vi "Connect.vi"(8 "error in (no error)":errorcluster, 9 "SQLITE3 open flags":u32(ring)=6 items=["SQLITE_OPEN_READONLY"=1, "SQLITE_OPEN_READWRITE"=2, "SQLITE_OPEN_CREATE"=4, "READWRITE | CREATE (default)"=6, "SQLITE_OPEN_DELETEONCLOSE"=8, "SQLITE_OPEN_EXCLUSIVE"=16, "SQLITE_OPEN_AUTOPROXY"=32, "SQLITE_OPEN_URI"=64, "SQLITE_OPEN_MEMORY"=128, "SQLITE_OPEN_MAIN_DB"=256, "SQLITE_OPEN_TEMP_DB"=512, "SQLITE_OPEN_TRANSIENT_DB"=1024, "SQLITE_OPEN_MAIN_JOURNAL"=2048, "SQLITE_OPEN_TEMP_JOURNAL"=4096, "SQLITE_OPEN_SUBJOURNAL"=8192, "SQLITE_OPEN_MASTER_JOURNAL"=16384, "SQLITE_OPEN_NOMUTEX"=32768, "SQLITE_OPEN_FULLMUTEX"=65536, "SQLITE_OPEN_SHAREDCACHE"=131072, "SQLITE_OPEN_PRIVATECACHE"=262144, "SQLITE_OPEN_WAL"=524288], 10 "path":string=":memory:") -> (0 "error out":errorcluster, 3 "SQLite3LV Connection out":refnum<class "sqlite3.lvclass">)   [LabVIEW 2014, in "SQLite3LV.lvlib" / "sqlite3.lvclass"]
doc: "Opens a connection to an SQLite3LV Connection database.\n\nThe path should be a valid URI resource or :memory:, an in-memory SQLite3 database.\n\nThe SQLITE3 Open Flags must be a valid combination of open flags. Use the OR primitive to combine flags. Incorrect open flags will likely result in SQLITE3 error 21 (library misuse).\n\nRefer to the documentation (sqlite3_open_v2()) for more information: https://www.sqlite.org/c3ref/open.html"
uses:
  sqlite3.lvclass
  sqlite3.lvclass/sqlite3.ctl
  SQLite3LV.lvlib
  sqlite3_64.dll
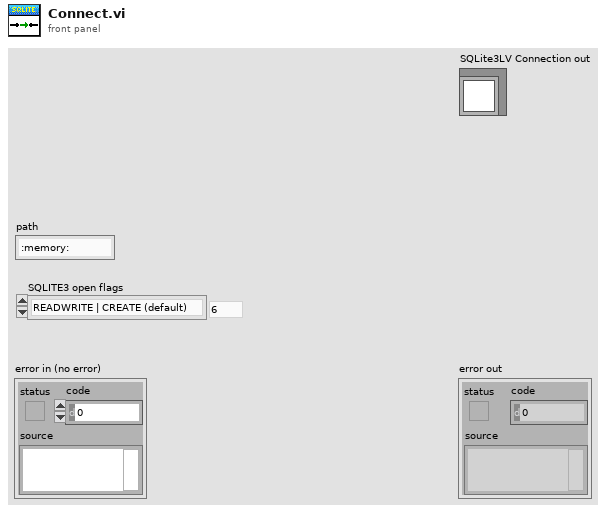
[diagram p1: front panel]
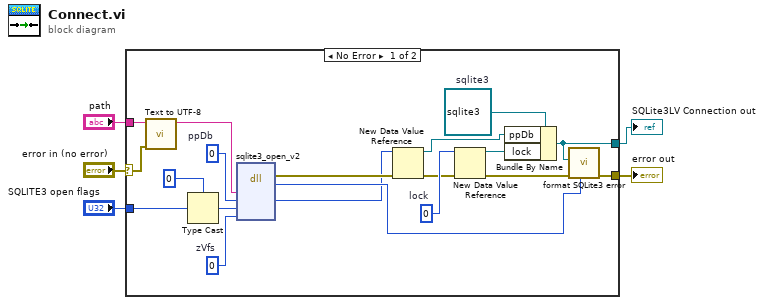
[diagram p0: block diagram]
diagram:
  n1 = case shown="No Error" "error in (no error)" {
    selector: "error in (no error)" -> [w15 w25]
    tunnel: [w6 w25] -> w4
    tunnel: "path" -> [w24 _]
    tunnel: "SQLITE3 open flags" -> [w19 _]
    tunnel: [w7 _] -> w1
    frame No Error {
      w14 = 0  # lock
      w16 = refnum<class "sqlite3.lvclass"> refnum  # sqlite3
      w20 = 0  # zVfs
      w21 = i64 0  # ppDb
      n2 = call "Text to UTF-8.vi"("error in"=w15, "text"=w24) -> ("utf-8 text"=w23:string)  [unwired: 8 in, 1 out]
      n3 = Type Cast(type=0 ("max queue size (-1, unlimited)"), x=w19) -> (*(type *) &x=w18:i32)
      n4 = dll-call lib="C:/Users/BobUser/Desktop/LVTables/sqlite3**.*" fn="sqlite3_open_v2"("path_utf8"=w23, "ppDb"=w21, "flags"=w18, "zVfs"=w20) -> (error out=w10:errorcluster, "return type"=w22:i32, "ppDb"=w8:i64)  [unwired: 6 in, 1 out]
      n5 = New Data Value Reference(data value=w8, error in=w10) -> (data value reference=w12:refnum<data-value>, error out=w11:errorcluster)
      n6 = New Data Value Reference(data value=w14, error in=w11) -> (data value reference=w13:refnum<data-value>, error out=w9:errorcluster)
      n7 = Bundle By Name(cluster=w16, "ppDb"=w12, "lock"=w13) -> (w7:refnum<class "sqlite3.lvclass">)
      n8 = call "format SQLite3 error.vi"("SQLite3LV Connection result"=w22, "error in (no error)"=w9, "psqlite"=w7) -> ("error out"=w6:errorcluster)  [unwired: 8 in]
    }
    frame Error {
    }
  }
  "error out" <- w4
  "SQLite3LV Connection out" <- w1
